vi "Set Parameters and data.vi"(8 "error in (no error)":errorcluster, 9 "Data":variant, 10 "Parameter":T1) -> (0 "error out":errorcluster)   [LabVIEW 2018, in "TTL IO.lvlib"]
doc: "Sends a parameters and data to the module. Can be either a full cluster of parameters or individual ones.\n_____\nCreated using Delacor QMH Event Scripter 4.2.1.88."
uses:
  TTL IO.lvlib
  Typedefs/CTL_Parameter_transfer_name.ctl
  Set Parameters and data Argument--cluster.ctl
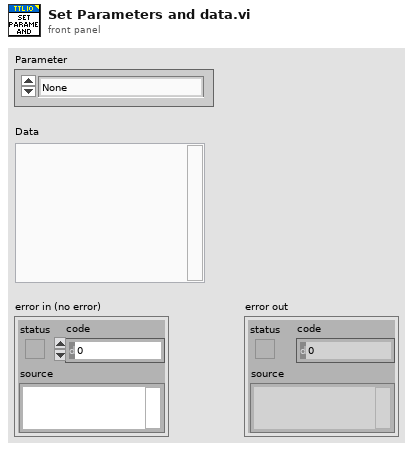
[diagram p1: front panel]
types:
  T1 = typedef "TTL IO.lvlib/CTL_Parameter_transfer_name.ctl" = enum16{"None", "All parameters", "IO parameters", "Conditions"}
  T2 = typedef "TTL IO.lvlib/Set Parameters and data Argument--cluster.ctl" = cluster{"Parameter":T1, "Data":variant}
  T3 = typedef "TTL IO.lvlib/Request Events--cluster.ctl" = cluster{"Stop Module":refnum<user-event>, "Show Panel":refnum<user-event>, "Hide Panel":refnum<user-event>, "Get Module Execution Status":refnum<user-event>, "Show Diagram":refnum<user-event>, "Set Parameters and data":refnum<user-event>}
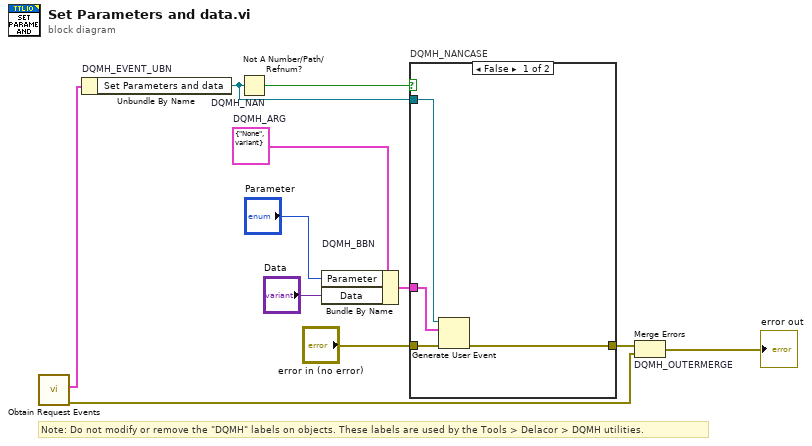
[diagram p0: block diagram]
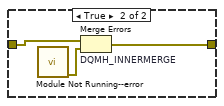
[diagram p2: hidden frame]
diagram:
  w5 = T2 {"Parameter"=enum."None", "Data"=variant}  # DQMH_ARG
  # "Note: Do not modify or remove the \"DQMH\" labels on objects. These labels are used by the Tools > Delacor > DQMH utilities."
  n1 = call "Obtain Request Events.vi"() -> ("error out"=w2:errorcluster, "TTL IO Request Events"=w1:T3)  [unwired: 10 in]
  n2 = Unbundle By Name "DQMH_EVENT_UBN"(w1) -> ("Set Parameters and data"=w7:refnum<user-event>)
  n3 = Not A Number/Path/Refnum? "DQMH_NAN"(number/path/refnum=w7) -> (NaN/Path/Refnum?=w8:bool)
  n4 = Bundle By Name "DQMH_BBN"(cluster=w5, "Parameter"="Parameter", "Data"="Data") -> (w9:T2)
  n5 = case "DQMH_NANCASE" shown="False" w8 {
    tunnel: "error in (no error)" -> [w15 w18]
    tunnel: [w14 w17] -> w6
    tunnel: w7 -> [w13 _]
    tunnel: w9 -> [w12 _]
    frame False {
      n6 = Generate User Event(user event=w13, event data cluster=w12, error in=w15) -> (error out=w14:errorcluster)  [unwired: 1 in, 1 out]
    }
    frame True {
      n7 = call "Module Not Running--error.vi"() -> ("error out"=w16:errorcluster)  [unwired: 11 in]
      n8 = Merge Errors "DQMH_INNERMERGE"(w18, w16) -> (w17:errorcluster)
    }
  }
  n9 = Merge Errors "DQMH_OUTERMERGE"(w6, w2) -> (→"error out":errorcluster)
